vi "Add Entire Hierarchy To Set.vi"(10 "Test Name":string, 11 "Set in":set{string}(c389)) -> (3 "Set out":set{string}(c389))   [LabVIEW 2020, in "Result Model.lvclass"]
uses:
  Result Model.lvclass
  Result Model.lvclass/Result Model.ctl
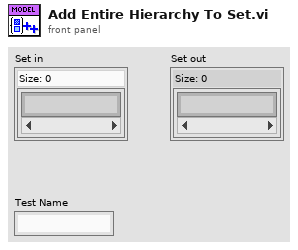
[diagram p1: front panel]
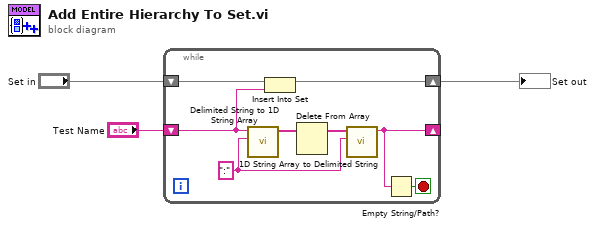
[diagram p0: block diagram]
diagram:
  n1 = while {
    shift-right: [w10] -> w2
    shift-left: "Set in" -> [w11]
    shift-right: [w4] -> _
    shift-left: "Test Name" -> [w6]
    stop <- w5 stop-if-true
    w8 = ":" ("delimiter")
    n2 = call <vilib>:"Delimited String to 1D String Array.vi"("delimiter"=w8, "delimited string"=w6) -> ("string array"=w9:string[])  [unwired: 9 in]
    n3 = Insert Into Set(10:w6, 11:w11) -> (3:w10:set{string})  [unwired: 1 out]
    n4 = Delete From Array(array=w9) -> (array with subset deleted=w7:string[])  [unwired: 2 in, 1 out]
    n5 = call <vilib>:"1D String Array to Delimited String.vi"("delimiter"=w8, "string array"=w7) -> ("delimited string"=w4:string)  [unwired: 9 in]
    n6 = Empty String/Path?(string/path=w4) -> (empty?=w5:bool)
  }
  "Set out" <- w2
